vi "SwissSPAD Live_Check Gate Definition Authorizaton.vi"(8 "Error In":errorcluster, 9 "OldVal":variant, 10 "NewVal":variant, 11 "Control Refnum":refnum<vi>) -> (0 "Error Out":errorcluster, 1 "Change Accepted?":bool, 2 "NewVal":variant, 3 "Control Refnum":refnum<vi>)   [LabVIEW 2021]
uses:
  SwissSPAD Live_SS3 DAQ Parameters.ctl
  SwissSPAD Live_SS3 Gate Definition.ctl
  SS3 Gate Width Definition Mode.ctl
  SwissSPAD Live_SS2 DAQ Parameters 3.ctl
  SwissSPAD Live_SS2 Gate Definition.ctl
  SwissSPAD Live_Globals.vi
panel:
  in  "SS3 DAQ Parameters":T1={"10 bits"=FALSE, "# Exposure Sequences"=0, "# 1-bit Frame per Gate"=255, "Gate Shift"=0, "# Gate Pairs per Set"=0, "# Sets"=1, "Laser Period"=0.0, "Sync Period"=0.0, "Gate Offset"=0, "Auto-adjust Gate Offset"=FALSE, "Gate Definition"={"gs_psincdec_0"=0, "gs_psincdec_1"=0, "gs_no_shift_adj_1"=0, "gate_adj_2"=0}, "Gate Width (ns)"=0.0, "Reversed Shift"=FALSE, "Intensity Mode"=FALSE, "Gate Definition Mode"=enum."Item 0"} {"Gate Width (ns)" min=0.0 max=100.0 format="%#_5g"; "# Sets" min=1}
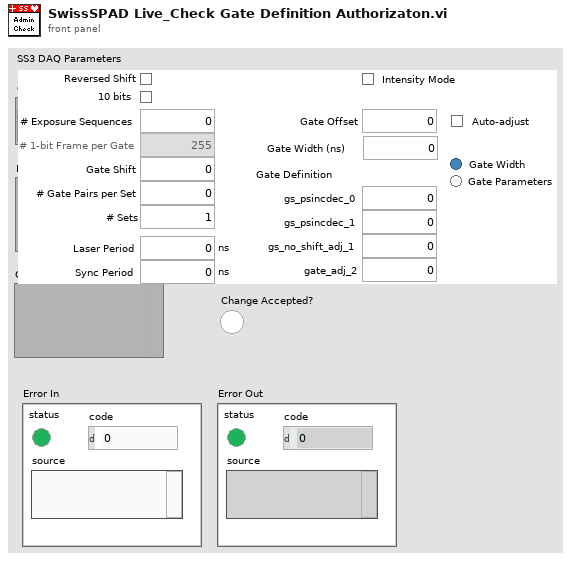
[diagram p1: front panel]
types:
  T1 = typedef "SwissSPAD Live_SS3 DAQ Parameters.ctl" = cluster{"10 bits":bool, "# Exposure Sequences":u32, "# 1-bit Frame per Gate":u32, "Gate Shift":u32, "# Gate Pairs per Set":u32, "# Sets":u32, "Laser Period":dbl[unit], "Sync Period":dbl[unit], "Gate Offset":u32, "Auto-adjust Gate Offset":bool, "Gate Definition":T2, "Gate Width (ns)":dbl, "Reversed Shift":bool, "Intensity Mode":bool, "Gate Definition Mode":T3}
  T2 = typedef "SwissSPAD Live_SS3 Gate Definition.ctl" = cluster{"gs_psincdec_0":u32, "gs_psincdec_1":u32, "gs_no_shift_adj_1":u32, "gate_adj_2":u32}
  T3 = typedef "SS3 Gate Width Definition Mode.ctl" = enum32{"Item 0", "Item 1"}
  T4 = typedef "SwissSPAD Live_SS2 DAQ Parameters 3.ctl" = cluster{"10 bits":bool, "# Exposure Sequences":u32, "# 1-bit Frame per Gate":u32, "Gate Shift":u32, "# Gates per Set":u32, "# Sets":u32, "Laser Period":dbl[unit], "Sync Period":dbl[unit], "Gate Offset":u32, "Auto-adjust Gate Offset":bool, "Gate Definition":T5, "Reversed Shift":bool}
  T5 = typedef "SwissSPAD Live_SS2 Gate Definition.ctl" = cluster{"gs_psincdec_0":u32, "gs_psincdec_1":u32, "gs_psincdec_2":u32, "gs_psincdec_3":u32, "gs_no_shift_adj_1":u32, "gs_no_shift_adj_2":u32, "gs_no_shift_adj_3":u32}
  T6 = cluster{"10 bits":bool, "# Exposure Sequences":bool, "# 1-bit Frame per Gate":bool, "Gate Shift":bool, "# Gates per Set":bool, "# Sets":bool, "Laser Period":bool, "Sync Period":bool, "Gate Offset":bool, "Auto-adjust Gate Offset":bool, "Gate Definition":cluster{"gs_psincdec_0":bool, "gs_psincdec_1":bool, "gs_psincdec_2":bool, "gs_psincdec_3":bool, "gs_no_shift_adj_1":bool, "gs_no_shift_adj_2":bool, "gs_no_shift_adj_3":bool}, "Reversed Shift":bool}
  T7 = cluster{"gs_psincdec_0":bool, "gs_psincdec_1":bool, "gs_psincdec_2":bool, "gs_psincdec_3":bool, "gs_no_shift_adj_1":bool, "gs_no_shift_adj_2":bool, "gs_no_shift_adj_3":bool}
  T8 = enum8{"Enabled", "Disabled", "Disabled and Grayed Out"}
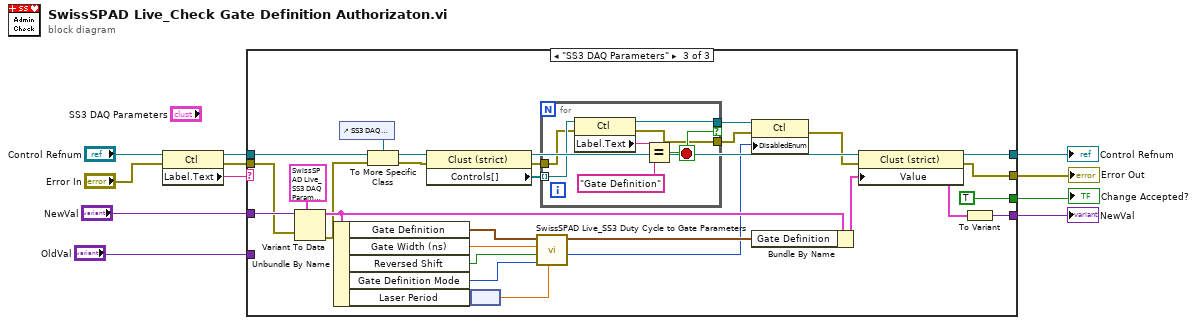
[diagram p0: block diagram]
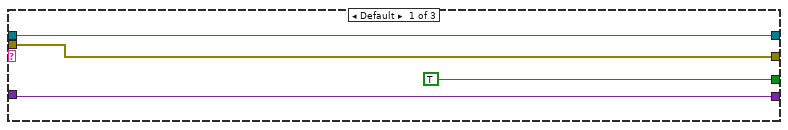
[diagram p2: hidden frame]
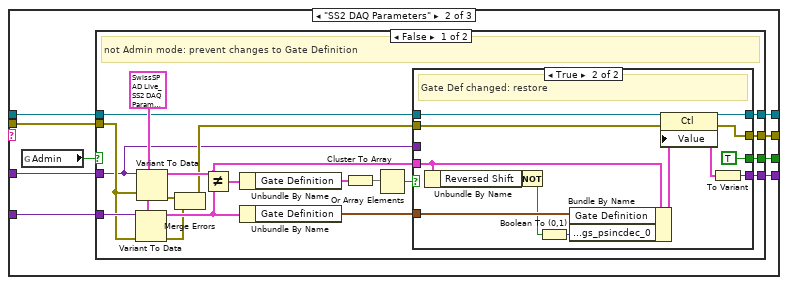
[diagram p3: hidden frame]
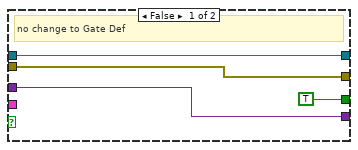
[diagram p4: hidden frame]
diagram:
  n1 = property class="Ctl"(reference="Control Refnum", error in="Error In") -> (reference out=w8:refnum<vi>, error out=w3:errorcluster, "Label.Text"=w9:string)
  n2 = case shown="\"SS3 DAQ Parameters\"" w9 {
    tunnel: w8 -> [w15 w23 w77]
    tunnel: [w15 w22 w91] -> w7
    tunnel: "NewVal" -> [w14 w21 w90]
    tunnel: [w14 w20 w64] -> w5
    tunnel: [w13 w18 w87] -> w4
    tunnel: w3 -> [w13 w17 w86]
    tunnel: [TRUE ("Change Accepted?") w19 TRUE] -> w2
    tunnel: "OldVal" -> [_ w16 _]
    frame Default {
    }
    frame "SS2 DAQ Parameters" {
      n3 = global read "SwissSPAD Live_Globals.vi" "Admin"() -> (w24:bool)
      n4 = case shown="False" w24 {
        selector: w24 -> [_ w61]
        tunnel: w23 -> [w33 w63]
        tunnel: [w32 w63] -> w22
        tunnel: w21 -> [w26 w62]
        tunnel: [w25 w62] -> w20
        tunnel: [w27 w61] -> w19
        tunnel: [w28 w60] -> w18
        tunnel: w17 -> [w42 w60]
        tunnel: w16 -> [w43 _]
        frame False {
          w41 = T4 {"10 bits"=FALSE, "# Exposure Sequences"=0, "# 1-bit Frame per Gate"=255, "Gate Shift"=0, "# Gates per Set"=0, "# Sets"=1, "Laser Period"=0.0, "Sync Period"=0.0, "Gate Offset"=0, "Auto-adjust Gate Offset"=FALSE, "Gate Definition"={"gs_psincdec_0"=0, "gs_psincdec_1"=0, "gs_psincdec_2"=0, "gs_psincdec_3"=0, "gs_no_shift_adj_1"=0, "gs_no_shift_adj_2"=0, "gs_no_shift_adj_3"=0}, "Reversed Shift"=FALSE} ("SS2 DAQ Parameters")
          # "not Admin mode: prevent changes to Gate Definition"
          n5 = Variant To Data(error in=w42, type=w41, Variant=w43) -> (data=w37:T4, error out=w30:errorcluster)
          n6 = Variant To Data(error in=w42, type=w41, Variant=w26) -> (data=w35:T4, error out=w31:errorcluster)
          n7 = Merge Errors(w31, w30) -> (w29:errorcluster)
          n8 = Not Equal?(x=w35, y=w37) -> (x != y?=w40:T6)
          n9 = Unbundle By Name(w40) -> ("Gate Definition"=w39:T7)
          n10 = Unbundle By Name(w37) -> ("Gate Definition"=w34:T5)
          n11 = Cluster To Array(cluster=w39) -> (array=w38:bool[])
          n12 = Or Array Elements(Boolean array=w38) -> (logical OR=w36:bool)
          n13 = case shown="True" w36 {
            tunnel: w35 -> [_ w52]
            tunnel: w34 -> [_ w59]
            tunnel: w33 -> [w47 w58]
            tunnel: [w47 w57] -> w32
            tunnel: w29 -> [w46 w56]
            tunnel: [w46 w55] -> w28
            tunnel: [TRUE TRUE] -> w27
            tunnel: w26 -> [w44 _]
            tunnel: [w44 w48] -> w25
            frame False {
              # "no change to Gate Def"
            }
            frame True {
              # "Gate Def changed: restore"
              n14 = Unbundle By Name(w52) -> ("Reversed Shift"=w51:bool)
              n15 = Not(x=w51) -> (.not. x?=w50:bool)
              n16 = Boolean To (0,1)(Boolean=w50) -> (0, 1=w49:i16)
              n17 = Bundle By Name(cluster=w52, "Gate Definition"=w59, "Gate Definition.gs_psincdec_0"=w49) -> (w54:T4)
              n18 = property class="Ctl"(reference=w58, error in=w56, "Value"=w54) -> (reference out=w57:refnum<vi>, error out=w55:errorcluster)
              n19 = To Variant(anything=w54) -> (Variant=w48:variant)
            }
          }
        }
        frame True {
          # "Admin mode: changes OK"
        }
      }
    }
    frame "SS3 DAQ Parameters" {
      n20 = Variant To Data(error in=w86, type=T1 {"10 bits"=FALSE, "# Exposure Sequences"=0, "# 1-bit Frame per Gate"=255, "Gate Shift"=0, "# Gate Pairs per Set"=0, "# Sets"=1, "Laser Period"=0.0, "Sync Period"=0.0, "Gate Offset"=0, "Auto-adjust Gate Offset"=FALSE, "Gate Definition"={"gs_psincdec_0"=0, "gs_psincdec_1"=0, "gs_no_shift_adj_1"=0, "gate_adj_2"=0}, "Gate Width (ns)"=0.0, "Reversed Shift"=FALSE, "Intensity Mode"=FALSE, "Gate Definition Mode"=enum."Item 0"} ("SS3 DAQ Parameters"), Variant=w90) -> (data=w84:T1, error out=w79:errorcluster)
      n21 = Unbundle By Name(w84) -> ("Gate Definition"=w67:T2, "Gate Width (ns)"=w68:dbl, "Reversed Shift"=w82:bool, "Gate Definition Mode"=w81:T3, "Laser Period"=w66:dbl[unit])
      n22 = control-ref of="SS3 DAQ Parameters"() -> (w75:refnum<vi>)
      n23 = To More Specific Class(target class=w75, reference=w77, error in=w79) -> (specific class reference=w76:refnum<vi>, error out=w78:errorcluster)
      n24 = property class="Clust (strict)"(reference=w76, error in=w78) -> (reference out=w80:refnum<vi>, error out=w72:errorcluster, "Controls[]"=w74:refnum<vi>[])
      n25 = node(w66) -> (w65:dbl)
      n26 = call "SwissSPAD Live_SS3 Duty Cycle to Gate Parameters.vi"("Period (ns)"=w65, "Gate Definition Mode"=w81, "Reversed Shift"=w82, "Gate Width (ns)"=w68, "Gate Definition in"=w67) -> ("Enabled State"=w69:T8, "Gate Definition out"=w83:T2)  [unwired: 5 in]
      n27 = for {
        tunnel: w74 -> [w98] mode=indexing
        tunnel: [w95] -> w73 if=w94
        tunnel: w72 -> [w93]
        tunnel: [w92] -> w71
        stop <- w94 stop-if-true
        n28 = property class="Ctl"(reference=w98, error in=w93) -> (reference out=w95:refnum<vi>, error out=w92:errorcluster, "Label.Text"=w97:string)
        n29 = Equal?(x=w97, y="Gate Definition") -> (x = y?=w94:bool)
      }
      n30 = property class="Ctl"(reference=w73, error in=w71, "DisabledEnum"=w69) -> (error out=w70:errorcluster)  [unwired: 1 out]
      n31 = Bundle By Name(cluster=w84, "Gate Definition"=w83) -> (w89:T1)
      n32 = property class="Clust (strict)"(reference=w80, error in=w70, "Value"=w89) -> (reference out=w91:refnum<vi>, error out=w87:errorcluster)
      n33 = To Variant(anything=w89) -> (Variant=w64:variant)
    }
  }
  "NewVal" <- w5
  "Control Refnum" <- w7
  "Error Out" <- w4
  "Change Accepted?" <- w2
